vi "Popup VI error handler.vi"(9 "messages":string[](array[string]), 10 "errors":bool[](array[boolean]), 11 "Input names (use ; as a separator)":string) -> (3 "No error":bool)   [LabVIEW 2025]
uses:
  <vilib>/Utility/error.llb/Trim Whitespace One-Sided.vi
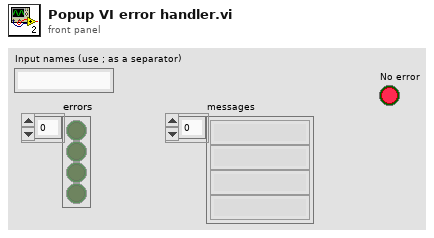
[diagram p1: front panel]
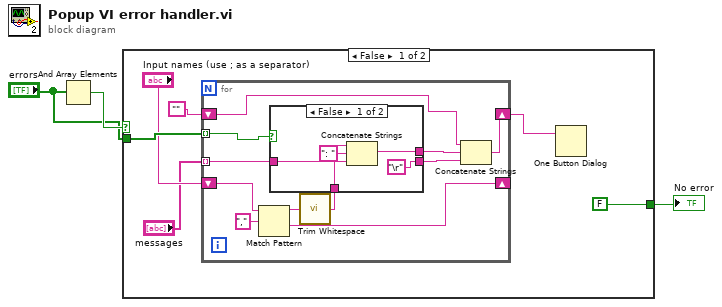
[diagram p0: block diagram]
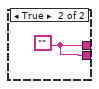
[diagram p2: hidden frame]
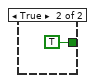
[diagram p3: hidden frame]
diagram:
  n1 = And Array Elements(Boolean array="errors") -> (logical AND=w3:bool)
  n2 = case shown="False" w3 {
    tunnel: "errors" -> [w9 _]
    tunnel: [FALSE ("force re-input?") TRUE ("force re-input?")] -> w1
    frame False {
      n3 = for {
        tunnel: w9 -> [w20] mode=indexing
        shift-right: [w17] -> _
        shift-left: "Input names (use ; as a separator)" -> [w18]
        tunnel: "messages" -> [w15] mode=indexing
        shift-right: [w14] -> w5
        shift-left: "" -> [w13]
        n4 = Match Pattern(string=w18, regular expression=",") -> (before substring=w16:string, after substring=w17:string)  [unwired: 1 in, 2 out]
        n5 = call <vilib>:"Trim Whitespace.vi"("string"=w16) -> ("trimmed string"=w10:string)  [unwired: 1 in]
        n6 = case shown="False" w20 {
          tunnel: w10 -> [w25 _]
          tunnel: w15 -> [w24 _]
          tunnel: [w23 w26] -> w12
          tunnel: ["\r" w26] -> w11
          frame False {
            n7 = Concatenate Strings(w25, ": " ("string"), w24) -> (w23:string)
          }
          frame True {
            w26 = ""
          }
        }
        n8 = Concatenate Strings(w13, w12, w11) -> (w14:string)
      }
      n9 = One Button Dialog(message=w5) -> ()  [unwired: 1 in, 1 out]
    }
    frame True {
    }
  }
  "No error" <- w1
